vi "Z900_navX_Util_DecodeProtocol_SignedThousandths.vi"(1 "Little Endian":u8[](array[numeric])) -> (0 "Signed Thousandths (0.000)":dbl[](array[numeric]))   [LabVIEW 2016, in "navX Library v2.lvlib"]
uses:
  navX Library v2.lvlib
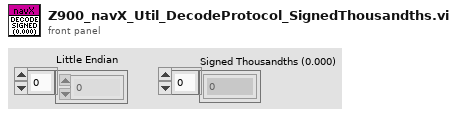
[diagram p1: front panel]
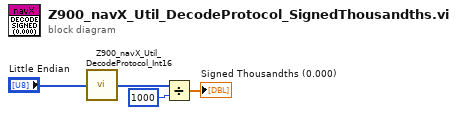
[diagram p0: block diagram]
diagram:
  n1 = call "Z900_navX_Util_DecodeProtocol_Int16.vi"("Little Endian"="Little Endian") -> ("Int16"=w3:i16[])
  n2 = Divide(x=w3, y=1000) -> (x/y=→"Signed Thousandths (0.000)":dbl[])
